vi "ROI entry screen-Adjust to correct times.vi"(8 "error in (no error)":errorcluster) -> (0 "error out":errorcluster, 2 "Corrected":bool)   [LabVIEW 2017]
uses:
  Globals/gl_ROI Entry UI globals.vi
  Global Variables/General Globals.vi
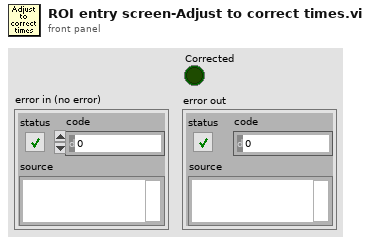
[diagram p1: front panel]
types:
  T1 = enum8{"Enabled", "Disabled", "Disabled and Grayed Out"}
  T2 = typedef "ROI entry screen ctrl refs cluster.ctl" = cluster{"Done button":refnum<vi>, "Imaging button":refnum<vi>, "Acquisition button":refnum<vi>, "POI dwell time (us)":refnum<vi>, "Scan dwell time per pixel (us)":refnum<vi>, "# of planes":refnum<vi>, "Zoom Ctrl":refnum<vi>, "Equal size":refnum<vi>, "Channel":refnum<vi>, "Image Display":refnum<vi>, "Z-Plane Selector":refnum<vi>, "Number of lines left":refnum<vi>, "Z-stack folder path":refnum<vi>, "POI Density":refnum<vi>, "Arb Plane Entry":refnum<vi>, "Whole plane":refnum<vi>, "Clear Last":refnum<vi>, "Clear All":refnum<vi>, "Trial Length (sec)":refnum<vi>, "Palette Type":refnum<vi>, "Intensity slider":refnum<vi>, "# POI":refnum<vi>, "Max Z Proj":refnum<vi>, "Zplane ind":refnum<vi>, "Wavelength (nm)":refnum<vi>, "Number of Trials":refnum<vi>, "Funct stim.trig.enable":refnum<vi>, "Funct stim.trig.delay (s)":refnum<vi>, "Line Mode":refnum<vi>, "Step size (µm)":refnum<vi>, "ROI move mode":refnum<vi>, "Cool-down time (s)":refnum<vi>, "Enable cool-down time":refnum<vi>, "Motor Z ind. (um)":refnum<vi>, "AOL Z ind. (um)":refnum<vi>, "Load Reference Image":refnum<vi>}
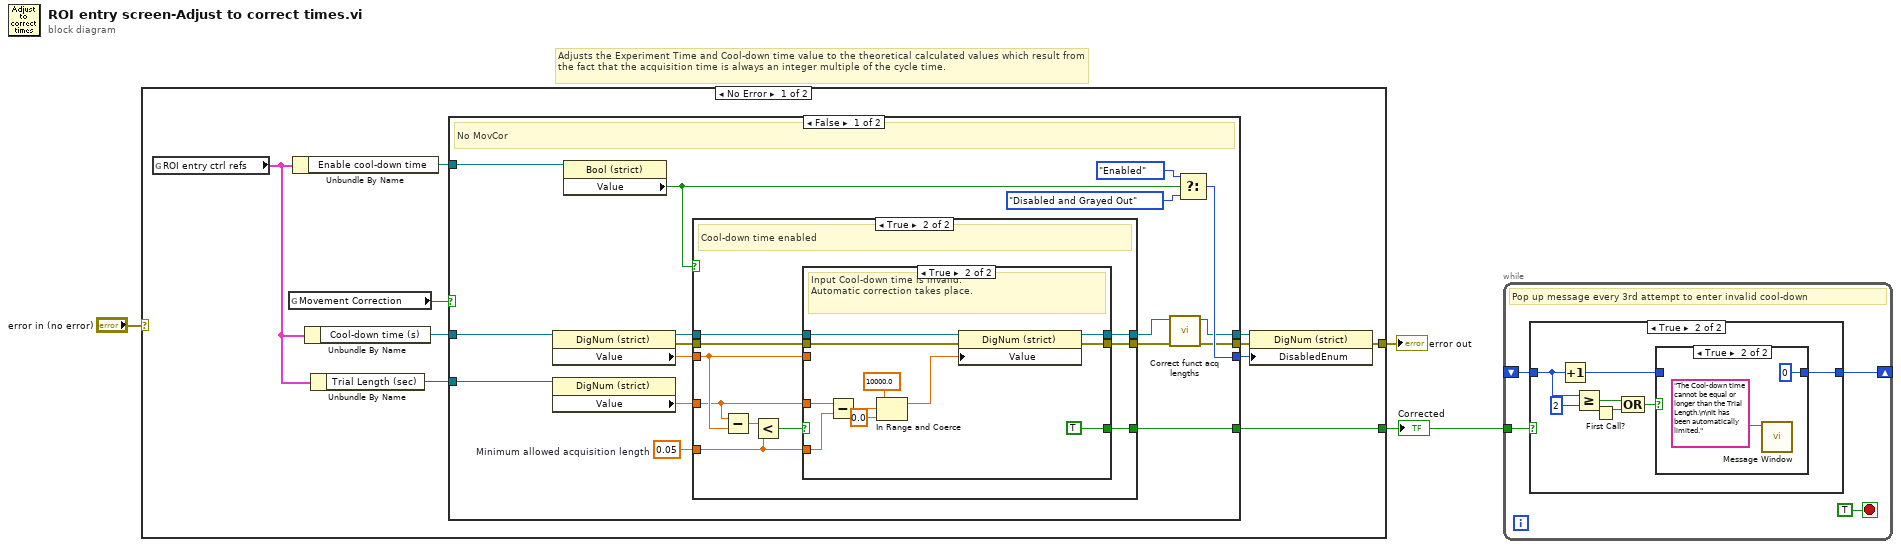
[diagram p0: block diagram]
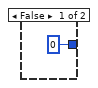
[diagram p2: hidden frame]
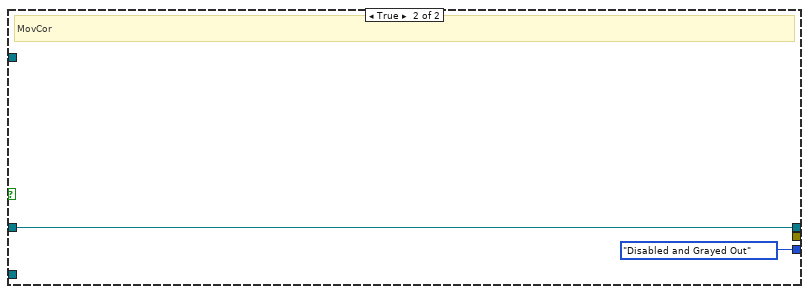
[diagram p6: hidden frame]
diagram:
  # "Adjusts the Experiment Time and Cool-down time value to the theoretical calculated values which result from the fact that the acquisition time is always an integer multiple of the cycle time."
  n1 = case shown="No Error" "error in (no error)" {
    selector: "error in (no error)" -> [_ w58]
    tunnel: [w8 w58] -> w3
    tunnel: [w7 _] -> w1
    frame No Error {
      n2 = global read "gl_ROI Entry UI globals.vi" "ROI entry ctrl refs"() -> (w9:T2)
      n3 = global read "General Globals.vi" "Movement Correction"() -> (w4:bool)
      n4 = Unbundle By Name(w9) -> ("Enable cool-down time"=w13:refnum<vi>)
      n5 = Unbundle By Name(w9) -> ("Cool-down time (s)"=w12:refnum<vi>)
      n6 = Unbundle By Name(w9) -> ("Trial Length (sec)"=w10:refnum<vi>)
      n7 = case shown="False" w4 {
        tunnel: w13 -> [w30 _]
        tunnel: w12 -> [w29 w56]
        tunnel: [w28 T1."Disabled and Grayed Out" ("Disabled")] -> w11
        tunnel: w10 -> [w25 _]
        tunnel: [w19 _] -> w7
        tunnel: [w15 w56] -> w6
        tunnel: [w14 _] -> w5
        frame False {
          w20 = 0.05  # Minimum allowed acquisition length
          # "No MovCor"
          n8 = property on="Property Node" class="DigNum (strict)"(reference=w29) -> (reference out=w24:refnum<vi>, error out=w23:errorcluster, "Value"=w22:dbl)  [unwired: 1 in]
          n9 = property on="Property Node" class="DigNum (strict)"(reference=w25) -> ("Value"=w21:dbl)  [unwired: 1 in, 2 out]
          n10 = property on="Property Node" class="Bool (strict)"(reference=w30) -> ("Value"=w18:bool)  [unwired: 1 in, 2 out]
          n11 = case shown="True" w18 {
            tunnel: w24 -> [w31 w40]
            tunnel: w23 -> [w32 w39]
            tunnel: w22 -> [_ w38]
            tunnel: [w31 w37] -> w16
            tunnel: [w32 w36] -> w17
            tunnel: w21 -> [_ w35]
            tunnel: w20 -> [_ w34]
            tunnel: [_ w33] -> w19
            frame False {
              # "Cool-down time disabled."
            }
            frame True {
              # "Cool-down time enabled"
              n12 = Subtract(x=w35, y=w38) -> (x-y=w42:dbl)
              n13 = Less?(x=w42, y=w34) -> (x < y?=w41:bool)
              n14 = case shown="True" w41 {
                tunnel: w40 -> [w43 w55]
                tunnel: w39 -> [w44 w54]
                tunnel: w38 -> [_ _]
                tunnel: [w43 w53] -> w37
                tunnel: [w44 w52] -> w36
                tunnel: w35 -> [_ w51]
                tunnel: w34 -> [_ w50]
                tunnel: [_ TRUE] -> w33
                frame False {
                  # "Input Cool-down time is valid"
                }
                frame True {
                  # "Input Cool-down time is invalid.\nAutomatic correction takes place."
                  n15 = Subtract(x=w51, y=w50) -> (x-y=w49:dbl)
                  n16 = In Range and Coerce(upper limit=10000.0, x=w49, lower limit=0.0) -> (coerced(x)=w46:dbl)  [unwired: 1 out]
                  n17 = property on="Property Node" class="DigNum (strict)"(reference=w55, error in=w54, "Value"=w46) -> (reference out=w53:refnum<vi>, error out=w52:errorcluster)
                }
              }
            }
          }
          n18 = call "Correct funct acq lengths.vi"("error in (no error)"=w17, "Cool-down time (s)"=w16) -> ("error out"=w14:errorcluster, "Cool-down time (s)"=w15:refnum<vi>)  [unwired: 7 in, 1 out]
          n19 = Select(t=T1."Enabled" ("Disabled"), s=w18, f=T1."Disabled and Grayed Out" ("Disabled")) -> (s? t:f=w28:T1)
        }
        frame True {
          # "MovCor"
        }
      }
      n20 = property on="Property Node" class="DigNum (strict)"(reference=w6, error in=w5, "DisabledEnum"=w11) -> (error out=w8:errorcluster)  [unwired: 1 out]
    }
    frame Error {
    }
  }
  "error out" <- w3
  "Corrected" <- w1
  n21 = while {
    shift-right: [w59] -> _
    shift-left: _ -> [w61]
    tunnel: w1 -> [w60]
    stop <- TRUE stop-if-true
    # "Pop up message every 3rd attempt to enter invalid cool-down"
    n22 = case shown="True" w60 {
      tunnel: w61 -> [_ w65]
      tunnel: [0 w66] -> w59
      frame False {
      }
      frame True {
        n23 = Increment(x=w65) -> (x+1=w67:i32)
        n24 = Greater Or Equal?(x=w65, y=2) -> (x >= y?=w68:bool)
        n25 = First Call?() -> (First Call?: T/F=w70:bool)
        n26 = Compound Arithmetic op=OR(w68, w70) -> (w69:bool)
        n27 = case shown="True" w69 {
          tunnel: w67 -> [w71 _]
          tunnel: [w71 0] -> w66
          frame False {
          }
          frame True {
            n28 = call "Message Window.vi"("Message string"="The Cool-down time cannot be equal or longer than the Trial Length.\n\nIt has been automatically limited.") -> ()  [unwired: 10 in, 1 out]
          }
        }
      }
    }
  }
